vi "NI_FPGA_PPG.contents.vi"() -> ()   [LabVIEW 2014, in "NI_FPGA_PPG.lvlib"]
doc: "loads all VIs into memory - required for building an application"
uses:
  NI_FPGA_PPG.lvlib
panel:
  out "error out":errorcluster
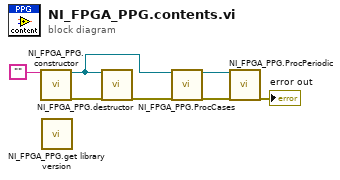
[diagram p0: block diagram]
diagram:
  n1 = call "NI_FPGA_PPG.constructor.vi"("name"="") -> ("i ref out"=w6:refnum<vi>, "error out"=w5:errorcluster)  [unwired: 16 in, 1 out]
  n2 = call "NI_FPGA_PPG.get library version.vi"() -> ()  [unwired: 1 in, 1 out]
  n3 = call "NI_FPGA_PPG.destructor.vi"("i ref in"=w6, "error in (no error)"=w5) -> ("error out"=w4:errorcluster)  [unwired: 17 in]
  n4 = call "NI_FPGA_PPG.ProcCases.vi"("i ref in"=w6, "error in (no error)"=w4) -> ("i ref out"=w3:refnum<vi>, "error out"=w2:errorcluster)  [unwired: 15 in, 1 out]
  n5 = call "NI_FPGA_PPG.ProcPeriodic.vi"("i ref in"=w3, "error in (no error)"=w2) -> ("error out"=→"error out":errorcluster)  [unwired: 15 in, 2 out]
